vi "DOE Final RMC.vi"(8 "error in (no error)":errorcluster) -> (0 "error out":errorcluster, 3 "Final Weight Output":T1)   [LabVIEW 2016]
uses:
  Utility/Custom Pallet Controls/Custom Pallet Forward.ctl
  Utility/Custom Pallet Controls/Custom Pallet String.ctl
panel:
  in  "Final Weight":T1
  in  "Complete":T2
  out "Front Program Name":string="Final Weight"
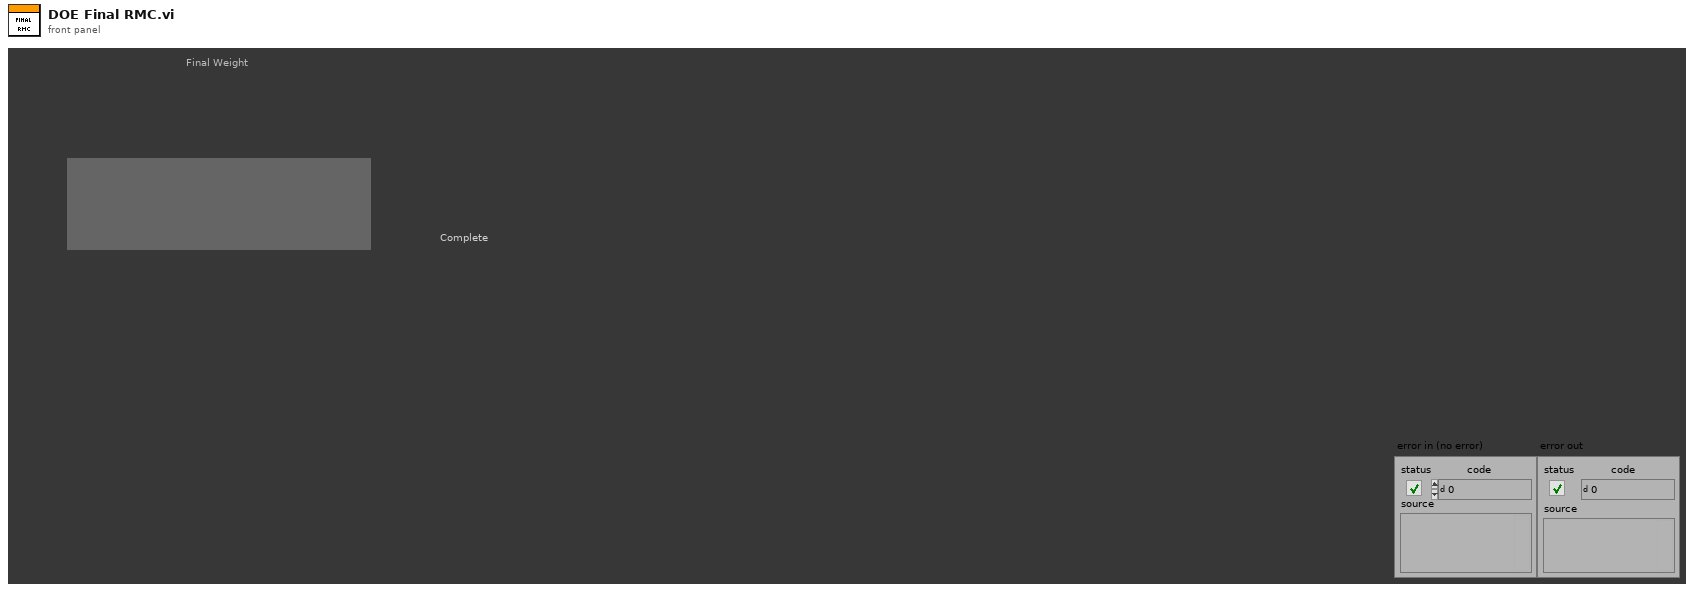
[diagram p1: front panel]
types:
  T1 = typedef "Custom Pallet String.ctl" = string
  T2 = typedef "Custom Pallet Forward.ctl" = bool
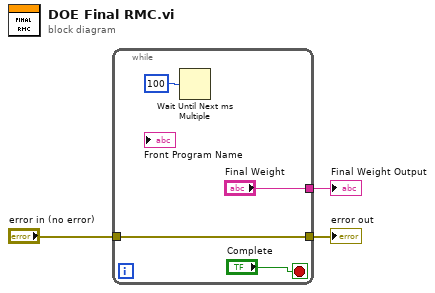
[diagram p0: block diagram]
diagram:
  n1 = while {
    tunnel: ["Final Weight"] -> w3
    tunnel: "error in (no error)" -> [w4]
    tunnel: [w4] -> w1
    stop <- "Complete" stop-if-true
    n2 = Wait Until Next ms Multiple(millisecond multiple=u32 100) -> ()  [unwired: 1 out]
  }
  "Final Weight Output" <- w3
  "error out" <- w1
